vi "get view class name.vi"(8 "error in":errorcluster, 11 "configuration in":refnum<class "NISE_CEF_serializable configuration.lvclass">) -> (0 "error out":errorcluster, 2 "view class":string, 3 "configuration out":refnum<class "NISE_CEF_serializable configuration.lvclass">)   [LabVIEW 2013, in "NISE_CEF_serializable configuration.lvclass"]
uses:
  NISE_CEF_serializable configuration.lvclass
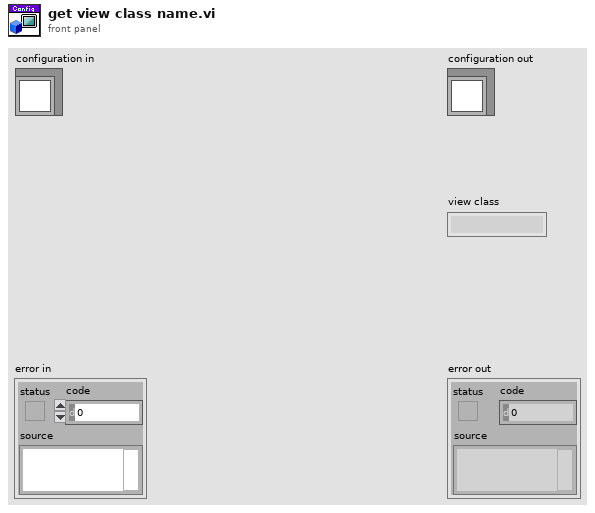
[diagram p1: front panel]
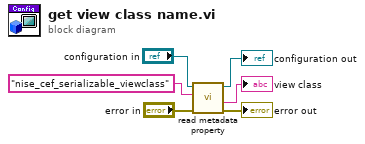
[diagram p0: block diagram]
diagram:
  n1 = call "read metadata property.vi"("error in"="error in", "key"="nise_cef_serializable_viewclass", "configuration in"="configuration in") -> ("error out"=→"error out":errorcluster, "value"=→"view class":string, "configuration out"=→"configuration out":refnum<class "NISE_CEF_serializable configuration.lvclass">)  [unwired: 5 in, 1 out]
